vi "R1_Calibrate DO.vi"() -> ()   [LabVIEW 2016]
uses:
  R2 Reactor Status v1.ctl
  <vilib>/Analysis/NI_AALPro.lvlib
panel:
  out "Intercept":dbl
  out "Slope":dbl
  in  "DO (mg/L)":dbl
  out "XY Graph":cluster{"Y":dbl[], "Y":dbl[]}[](graph)
  in  "Begin Calibration":bool
  in  "Number of Calibration Points":i32=3
  out "DO Amperage":dbl
  in  "Acquire":bool
  # "After bubbling N2 through flask for 3-5 minutes, DO concentration is 0 mg/L\n\nAfter bubbling air through flask for 3-5 minutes, DO concentration is:\n8.24 mg/L @ 25 C\n9.08 mg/L @  20C"
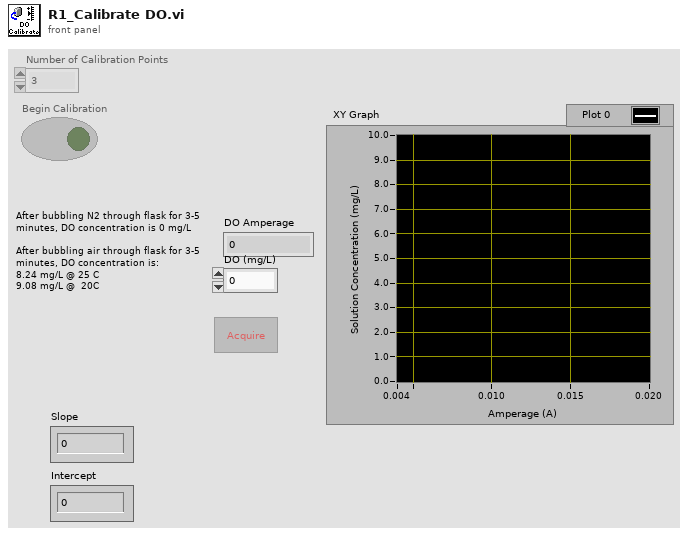
[diagram p1: front panel]
types:
  T1 = enum8{"Enabled", "Disabled", "Disabled and Grayed Out"}
  T2 = typedef "R2Variables.lvlib/R2 Reactor Status v1.ctl" = cluster{"Water Pump":bool, "Media Pump":bool, "Effluent Pump":bool, "Base Pump":bool, "Gas Pump":bool, "Acid Pump":bool, "Air Release Valve":bool, "N2 Valve":bool, "pH":dbl, "DO (mg/L)":dbl, "pH Amp (A)":dbl, "DO Amp (A)":dbl, "Release Flow":dbl, "Compressed Air":dbl, "Reactor Status":sgl, "Air Valve":bool}
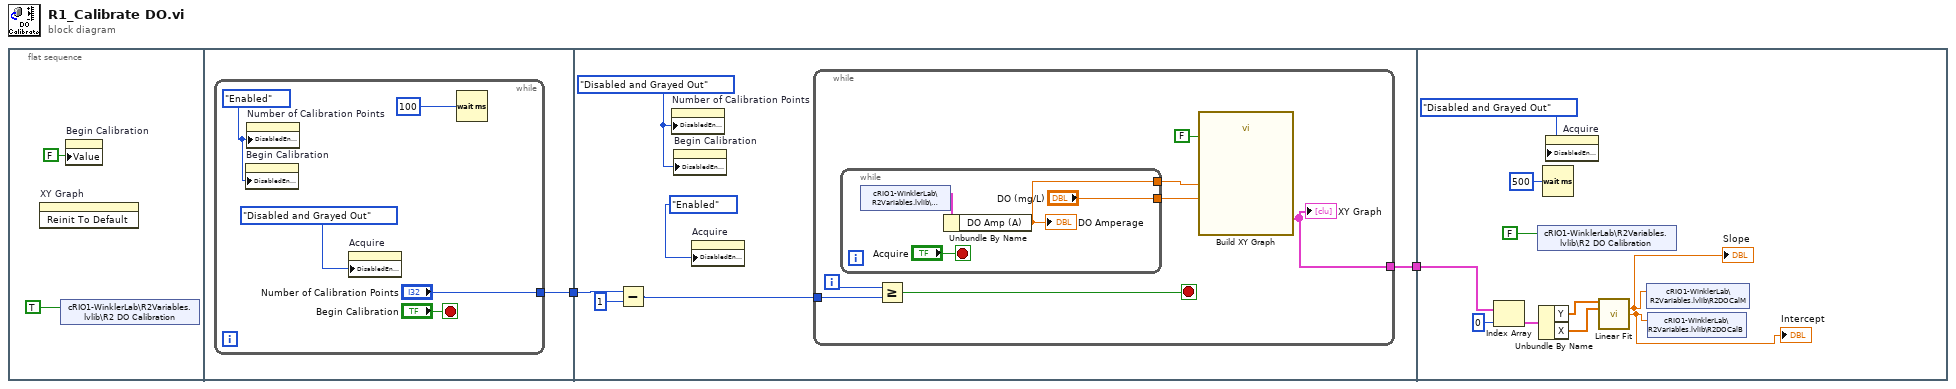
[diagram p0: block diagram]
diagram:
  n1 = flat-sequence {
    tunnel: [w5] -> w2
    tunnel: w2 -> [w13]
    tunnel: [w14] -> w1
    tunnel: w1 -> [w36]
    frame #0 {
      n2 = invoke on="XY Graph" class="XYGraph (strict)" method="Reinit To Default"() -> ()  [unwired: 3 in, 3 out]
      n3 = shared-variable "cRIO1-WinklerLab\\R2Variables.lvlib\\R2 DO Calibration"(TRUE ("Calibrating")) -> ()  [unwired: 1 in, 1 out]
      n4 = property on="Begin Calibration" class="Bool (strict)"("Value"=FALSE ("Begin Calibration")) -> ()  [unwired: 2 in, 2 out]
    }
    frame #1 {
      n5 = while {
        tunnel: ["Number of Calibration Points"] -> w5
        stop <- "Begin Calibration" stop-if-true
        w6 = T1."Enabled" ("Disabled")
        n6 = property on="Begin Calibration" class="Bool (strict)"("DisabledEnum"=w6) -> ()  [unwired: 2 in, 2 out]
        n7 = property on="Number of Calibration Points" class="DigNum (strict)"("DisabledEnum"=w6) -> ()  [unwired: 2 in, 2 out]
        n8 = property on="Acquire" class="Bool"("DisabledEnum"=T1."Disabled and Grayed Out" ("Disabled")) -> ()  [unwired: 2 in, 2 out]
        n9 = Wait (ms)(milliseconds to wait=u32 100) -> ()  [unwired: 1 out]
      }
    }
    frame #2 {
      w16 = T1."Disabled and Grayed Out" ("Disabled")
      n10 = Subtract(x=w13, y=1) -> (x-y=w11:i32)
      n11 = property on="Number of Calibration Points" class="DigNum (strict)"("DisabledEnum"=w16) -> ()  [unwired: 2 in, 2 out]
      n12 = property on="Begin Calibration" class="Bool (strict)"("DisabledEnum"=w16) -> ()  [unwired: 2 in, 2 out]
      n13 = property on="Acquire" class="Bool"("DisabledEnum"=T1."Enabled" ("Disabled")) -> ()  [unwired: 2 in, 2 out]
      n14 = while {
        tunnel: w11 -> [w19]
        tunnel: [w20] -> w14
        i -> [w22]
        stop <- w23 stop-if-true
        n15 = while {
          tunnel: [w26] -> w17
          tunnel: ["DO (mg/L)"] -> w18
          stop <- "Acquire" stop-if-true
          n16 = shared-variable "cRIO1-WinklerLab\\R2Variables.lvlib\\R2Status"() -> (w24:T2)  [unwired: 1 in, 1 out]
          n17 = Unbundle By Name(w24) -> ("DO Amp (A)"=w26:dbl)
          "DO Amperage" <- w26
        }
        n18 = Greater Or Equal?(x=w22, y=w19) -> (x >= y?=w23:bool)
        n19 = call "Build XY Graph"("Reset"=FALSE, "Y Input"=w18, "X Input"=w17) -> ("XY Graph"=w20:cluster{"X":dbl[], "Y":dbl[]}[])  [unwired: 7 in, 1 out]
        "XY Graph" <- w20
      }
    }
    frame #3 {
      n20 = Index Array(array=w36, index=0) -> (element=w34:cluster{"X":dbl[], "Y":dbl[]})
      n21 = shared-variable "cRIO1-WinklerLab\\R2Variables.lvlib\\R2 DO Calibration"(FALSE ("Calibrating")) -> ()  [unwired: 1 in, 1 out]
      n22 = Unbundle By Name(w34) -> ("Y"=w33:dbl[], "X"=w32:dbl[])
      n23 = Wait (ms)(milliseconds to wait=u32 500) -> ()  [unwired: 1 out]
      n24 = property on="Acquire" class="Bool"("DisabledEnum"=T1."Disabled and Grayed Out" ("Disabled")) -> ()  [unwired: 2 in, 2 out]
      n25 = call <vilib>:"Linear Fit.vi"("Y"=w33, "X"=w32) -> ("slope"=w29:dbl, "intercept"=w28:dbl)  [unwired: 9 in, 3 out]
      "Intercept" <- w28
      "Slope" <- w29
      n26 = shared-variable "cRIO1-WinklerLab\\R2Variables.lvlib\\R2DOCalM"(w29) -> ()  [unwired: 1 in, 1 out]
      n27 = shared-variable "cRIO1-WinklerLab\\R2Variables.lvlib\\R2DOCalB"(w28) -> ()  [unwired: 1 in, 1 out]
    }
  }
